vi "checkFinishNormalGamePlayVSS.vi"(8 "error in (no error)":errorcluster, 10 "Game in":refnum<class "Game.lvclass">, 11 "NormalGamePlayVSS in":refnum<class "NormalGamePlayVSS.lvclass">) -> (0 "error out":errorcluster, 2 "Boolean":bool, 3 "NormalGamePlayVSS out":refnum<class "NormalGamePlayVSS.lvclass">)   [LabVIEW 2023, in "NormalGamePlayVSS.lvclass"]
uses:
  NormalGamePlayVSS.lvclass
  Game_class/Game.lvclass
  Game_class/Game.lvclass/Game.ctl
  Events_class/Events.lvclass/Events.ctl
  Game_class/Read Referee.vi
  Game_class/Read EventsRef.vi
  Events_class/Read ball_out_of_vision.vi
  Events_class/Read ball_out.vi
  Referee_class/Referee.lvclass
  Events_class/Events.lvclass
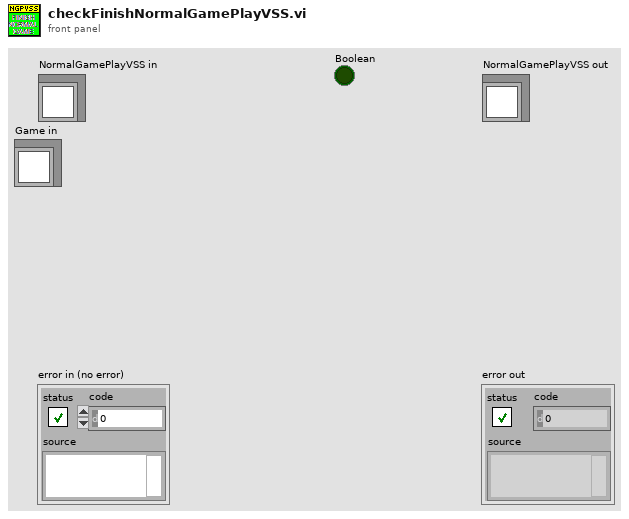
[diagram p1: front panel]
types:
  T1 = enum16{"AUTO", "GAME_ON", "STOP", "KICKOFF", "FREE_BALL", "GOAL_KICK", "PENALTY_KICK", "FREE_KICK"}
  T2 = typedef "Command.ctl" = enum16{"AUTO", "GAME_ON", "STOP", "HALT", "KICKOFF_ALLY", "KICKOFF_ENEMY", "FREE_BALL", "GOAL_KICK_ENEMY", "GOAL_KICK_ALLY", "PENALTY_KICK_ENEMY", "PENALTY_KICK_ALLY", "FREE_KICK"}
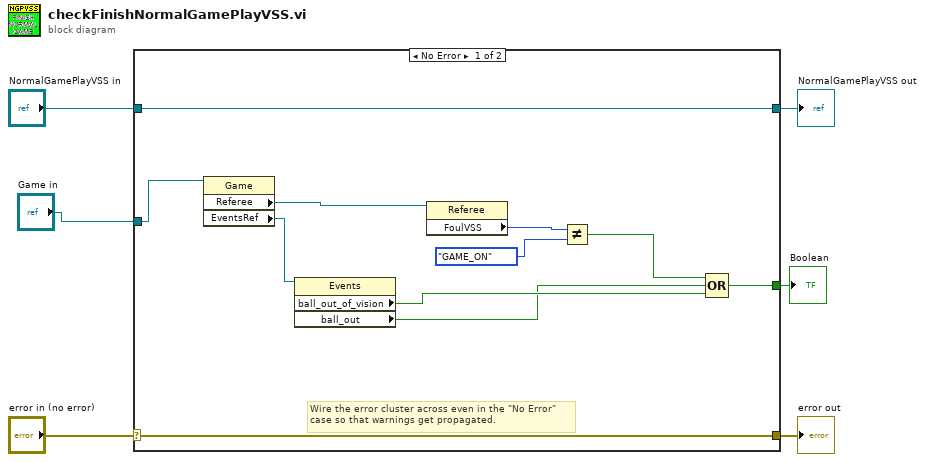
[diagram p0: block diagram]
diagram:
  n1 = case shown="No Error" "error in (no error)" {
    selector: "error in (no error)" -> [w16 w19]
    tunnel: [w16 w19] -> w5
    tunnel: [w17 w18] -> w3
    tunnel: "NormalGamePlayVSS in" -> [w17 w18]
    tunnel: "Game in" -> [w9 _]
    tunnel: [w8 _] -> w1
    frame No Error {
      # "Wire the error cluster across even in the \"No Error\"\ncase so that warnings get propagated."
      n2 = property class="Game"(reference=w9) -> ("Referee"=w15:refnum<class "Referee.lvclass">, "EventsRef"=w13:refnum<class "Events.lvclass">)  [unwired: 1 in, 2 out]
      n3 = property class="Events"(reference=w13) -> ("ball_out_of_vision"=w11:bool, "ball_out"=w10:bool)  [unwired: 1 in, 2 out]
      n4 = property class="Referee"(reference=w15) -> ("FoulVSS"=w14:T2)  [unwired: 1 in, 2 out]
      n5 = Not Equal?(x=w14, y=T1."GAME_ON") -> (x != y?=w12:bool)
      n6 = Compound Arithmetic op=OR(w12, w10, w11) -> (w8:bool)
    }
    frame Error {
    }
  }
  "error out" <- w5
  "NormalGamePlayVSS out" <- w3
  "Boolean" <- w1
